vi "enqMulti.vi"(8 "error in (no error)":errorcluster, 10 "array of cmds":T2(array[cluster]), 11 "eventcluster":T1) -> (0 "error out":errorcluster)   [LabVIEW 2017]
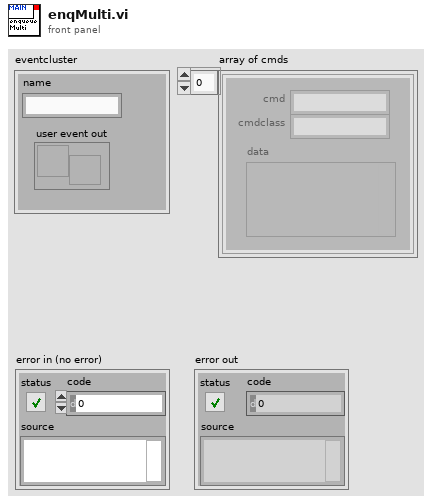
[diagram p1: front panel]
types:
  T1 = cluster{"name":string, "user event out":refnum<user-event>}
  T2 = cluster{"cmd":string, "cmdclass":string, "data":variant}[]
  T3 = cluster{"array of cmds":cluster{"cmd":string, "cmdclass":string, "data":variant}[]}
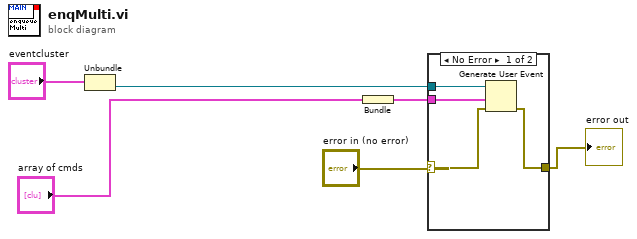
[diagram p0: block diagram]
diagram:
  n1 = Unbundle("eventcluster") -> ("user event out"=w4:refnum<user-event>)  [unwired: 1 out]
  n2 = Bundle("array of cmds"="array of cmds") -> (w2:T3)  [unwired: 1 in]
  n3 = case shown="No Error" "error in (no error)" {
    selector: "error in (no error)" -> [w9 w11]
    tunnel: w4 -> [w10 _]
    tunnel: [w8 w11] -> w5
    tunnel: w2 -> [w7 _]
    frame No Error {
      n4 = Generate User Event(user event=w10, event data cluster=w7, error in=w9) -> (error out=w8:errorcluster)  [unwired: 1 in, 1 out]
    }
    frame Error {
    }
  }
  "error out" <- w5
